vi "Remove Lower Percentile from Array.vi"(8 "Error In":errorcluster, 9 "Low Percentile to Reject":dbl, 11 "Array in":dbl[](array[numeric])) -> (0 "Error Out":errorcluster, 1 "# Rejected Elements":i32, 2 "Array Indices out":i32[](array[numeric]), 3 "(Sorted) Array out":dbl[](array[numeric]))   [LabVIEW 2021, in "Arrays.lvlib"]
uses:
  <userlib>/_OpenG.lib/array/array.llb/Sort 1D Array (DBL)__ogtk.vi
  <vilib>/gmath/statdist.llb/st_Percentiles (scalar).vi
  Arrays.lvlib
  <vilib>/gmath/NI_Gmath.lvlib
  Error/Error.lvlib
  <userlib>/_OpenG.lib/array/array.llb/openg_array.lvlib
panel:
  # "see the License on the block diagram (Ctrl+E or Window:Show Block Diagram)"
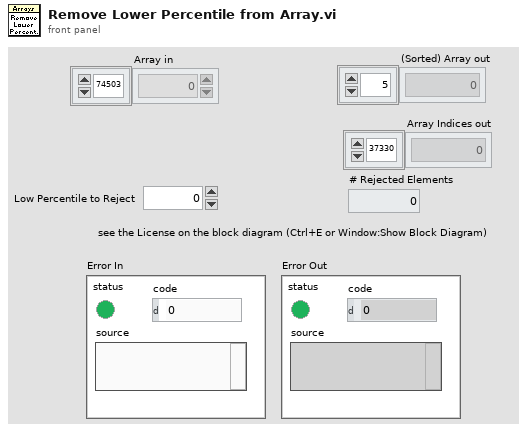
[diagram p1: front panel]
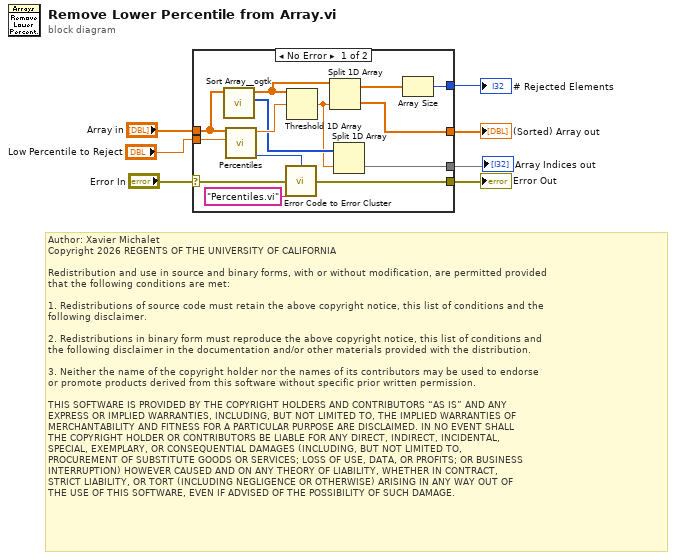
[diagram p0: block diagram]
diagram:
  # "Author: Xavier Michalet\nCopyright 2026 REGENTS OF THE UNIVERSITY OF CALIFORNIA\n\nRedistribution and use in source and binary forms, with or without modification, are permitted provided\nthat the following conditions are met:\n\n1. Redistributions of source code must retain the above copyright notice, this list of conditions and the\nfollowing disclaimer.\n\n2. Redistributions in binary form must reproduce the above copyright notice, this list of conditions and\nthe following disclaimer in the documentation and/or other materials provided with the distribution.\n\n3. Neither the name of the copyright holder nor the names of its contributors may be used to endorse \nor promote products derived from this software without specific prior written permission.\n\nTHIS SOFTWARE IS PROVIDED BY THE COPYRIGHT HOLDERS AND CONTRIBUTORS “AS IS” AND ANY \nEXPRESS OR IMPLIED WARRANTIES, INCLUDING, BUT NOT LIMITED TO, THE IMPLIED WARRANTIES OF\nMERCHANTABILITY AND FITNESS FOR A PARTICULAR PURPOSE ARE DISCLAIMED. IN NO EVENT SHALL\nTHE COPYRIGHT HOLDER OR CONTRIBUTORS BE LIABLE FOR ANY DIRECT, INDIRECT, INCIDENTAL, \nSPECIAL, EXEMPLARY, OR CONSEQUENTIAL DAMAGES (INCLUDING, BUT NOT LIMITED TO, \nPROCUREMENT OF SUBSTITUTE GOODS OR SERVICES; LOSS OF USE, DATA, OR PROFITS; OR BUSINESS\nINTERRUPTION) HOWEVER CAUSED AND ON ANY THEORY OF LIABILITY, WHETHER IN CONTRACT, \nSTRICT LIABILITY, OR TORT (INCLUDING NEGLIGENCE OR OTHERWISE) ARISING IN ANY WAY OUT OF\nTHE USE OF THIS SOFTWARE, EVEN IF ADVISED OF THE POSSIBILITY OF SUCH DAMAGE."
  n1 = case shown="No Error" "Error In" {
    selector: "Error In" -> [w19 w23]
    tunnel: "Low Percentile to Reject" -> [w21 _]
    tunnel: "Array in" -> [w16 w22]
    tunnel: [w20 w23] -> w4
    tunnel: [w13 w22] -> w3
    tunnel: [w11 _] -> w2
    tunnel: [w8 _] -> w1
    frame No Error {
      n2 = call-poly <userlib>:"Sort Array__ogtk.vi"("Array in"=w16) -> ("Sorted Pointers"=w10:i32[], "Sorted Array out"=w14:dbl[])  [unwired: 9 in]
      n3 = call-poly <vilib>:"Percentiles.vi"("p"=w21, "x array"=w16) -> ("error"=w18:i32, "percentile"=w15:dbl)  [unwired: 8 in]
      n4 = call "Error Code to Error Cluster.vi"("Error Code"=w18, "Error Source"="Percentiles.vi", "Error In"=w19) -> ("Error Out"=w20:errorcluster)  [unwired: 12 in]
      n5 = Threshold 1D Array(2:w15, 3:w14) -> (0:w9:dbl)  [unwired: 1 in]
      n6 = Split 1D Array(array=w14, index=w9) -> (first subarray=w12:dbl[], second subarray=w13:dbl[])
      n7 = Split 1D Array(array=w10, index=w9) -> (second subarray=w8:i32[])  [unwired: 1 out]
      n8 = Array Size(array=w12) -> (size(s)=w11:i32)
    }
    frame Error {
    }
  }
  "(Sorted) Array out" <- w3
  "# Rejected Elements" <- w2
  "Error Out" <- w4
  "Array Indices out" <- w1
